vi "Reset.vi"(8 "error in (no error)":errorcluster, 11 "PacificPowerSource in":refnum<class "PacificPowerSource.lvclass">) -> (0 "error out":errorcluster, 3 "PacificPowerSource out":refnum<class "PacificPowerSource.lvclass">)   [LabVIEW 2018, in "AcPwrPlugins.lvlib" / "PacificPowerSource.lvclass"]
doc: "This VI resets the instrument."
uses:
  PacificPowerSource.lvclass
  <instrlib>/Pacific Power UPC Series/Pacific Power UPC Series.lvlib
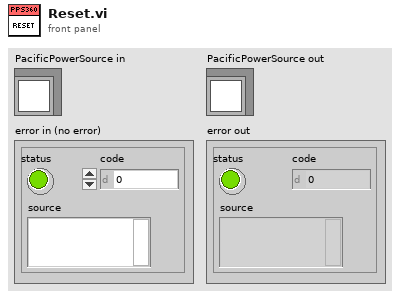
[diagram p1: front panel]
types:
  T1 = typedef "AcPwrPlugins.lvlib/PacificPowerSource.lvclass/DeviceSettings.ctl" = cluster{"Handle":string, "Connected":bool, "Clear Device (F)":bool, "btnIdQuery":bool, "btnReset":bool, "Program #":cluster{"Phase B (Degrees)":i32, "Waveform A (1: Sine)":i32, "Voltage Level (Va)":dbl, "Program Number (0)":i32, "Voltage Level (Vb) ":dbl, "Form (3: Three)":u16, "Coupling  (0: Direct)":u16, "Frequency (45Hz)":dbl, "Current Limit (40A)":dbl, "Phase C (Degrees)":i32, "Voltage Level (Vc)":dbl, "Waveform B (1: Sine)":i32, "Waveform C (1: Sine)":i32}[], "Impedance Parameters (off, 0.00)":cluster{"State":bool, "Impedance":dbl}, "Transient Execution (F)":bool, "OutputEnabled":bool, "Source Range":cluster{"Frequency Minimum (45 Hz)":dbl, "Frequency Maximum (1200 Hz)":dbl, "Voltage Maximum (V)":dbl, "Voltage Minimum (V)":dbl, "Range Control (0: Auto)":u16, "Initial Voltage (0V)":u16, "Frequency Range (600Hz)":u16}, "Port Type":enum16{"GPIB", "Serial"}}[]
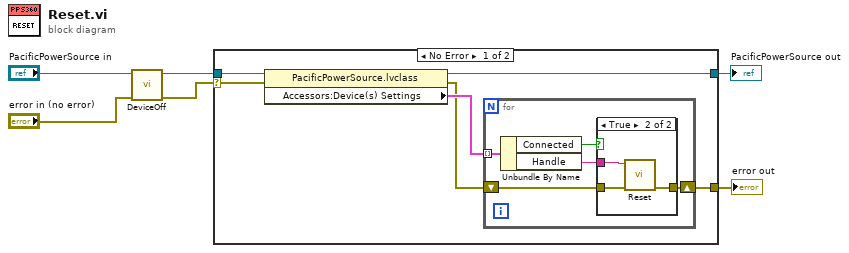
[diagram p0: block diagram]
diagram:
  n1 = call-dynamic "DeviceOff.vi"("error in (no error)"="error in (no error)", "PacificPowerSource in"="PacificPowerSource in") -> ("error out"=w3:errorcluster, "PacificPowerSource out"=w1:refnum<class "PacificPowerSource.lvclass">)  [unwired: 8 in]
  n2 = case shown="No Error" w3 {
    selector: w3 -> [w9 w22]
    tunnel: w1 -> [w10 w23]
    tunnel: [w8 w23] -> w6
    tunnel: [w7 w22] -> w5
    frame No Error {
      n3 = property class="PacificPowerSource.lvclass"(reference=w10, error in=w9) -> (reference out=w8:refnum<class "PacificPowerSource.lvclass">, error out=w11:errorcluster, "Accessors:Device(s) Settings"=w12:T1)
      n4 = for {
        tunnel: w12 -> [w17] mode=indexing
        shift-right: [w14] -> w7
        shift-left: w11 -> [w15]
        n5 = Unbundle By Name(w17) -> ("Connected"=w13:bool, "Handle"=w16:string)
        n6 = case shown="True" w13 {
          tunnel: w16 -> [_ w19]
          tunnel: w15 -> [w18 w21]
          tunnel: [w18 w20] -> w14
          frame False {
          }
          frame True {
            n7 = call <instrlib>:"Reset.vi"("error in (no error)"=w21, "VISA resource name"=w19) -> ("error out"=w20:errorcluster)  [unwired: 8 in, 1 out]
          }
        }
      }
    }
    frame Error {
    }
  }
  "error out" <- w5
  "PacificPowerSource out" <- w6
